vi "Log (2D).vi"(8 "error in (no error)":errorcluster, 10 "Log scale?":bool, 11 "Array in":dbl[][](array[numeric])) -> (0 "error out":errorcluster, 3 "Array out":dbl[][](array[numeric]))   [LabVIEW 2016, in "Retrieve and Visualize.lvclass"]
uses:
  Retrieve and Visualize.lvclass
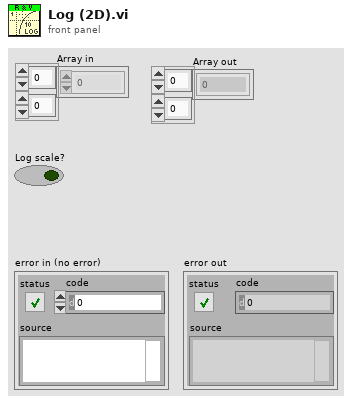
[diagram p1: front panel]
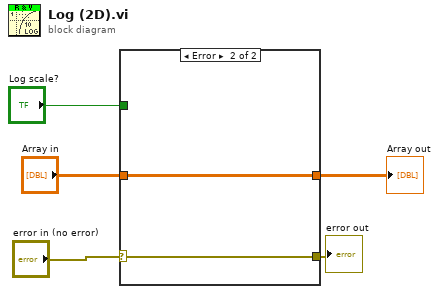
[diagram p0: block diagram]
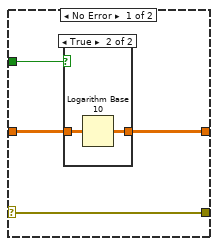
[diagram p2: hidden frame]
diagram:
  n1 = case shown="Error" "error in (no error)" {
    selector: "error in (no error)" -> [w6 w14]
    tunnel: [w9 w13] -> w5
    tunnel: "Log scale?" -> [w8 _]
    tunnel: "Array in" -> [w7 w13]
    tunnel: [w6 w14] -> w1
    frame No Error {
      n2 = case shown="True" w8 {
        tunnel: w7 -> [w10 w12]
        tunnel: [w10 w11] -> w9
        frame False {
        }
        frame True {
          n3 = Logarithm Base 10(1:w12) -> (0:w11:dbl[][])
        }
      }
    }
    frame Error {
    }
  }
  "Array out" <- w5
  "error out" <- w1
